vi "Convert_Midi_Data_To_Arduino.vi"() -> ()   [LabVIEW 2020]
uses:
  <vilib>/express/express arith-compare/Formula/XNode/ExpressFormulaBlockNode.xnode
panel:
  out "size(s)":i32
  out "String":string
  out "Array 3":dbl[](array[numeric])
  in  "Stop":bool
  out "x-y":dbl
  out "Array 2":i32[](array[numeric])
  out "Array":T1(array[cluster])
  out "value":T2(array[cluster])
  in  "JSON string":string
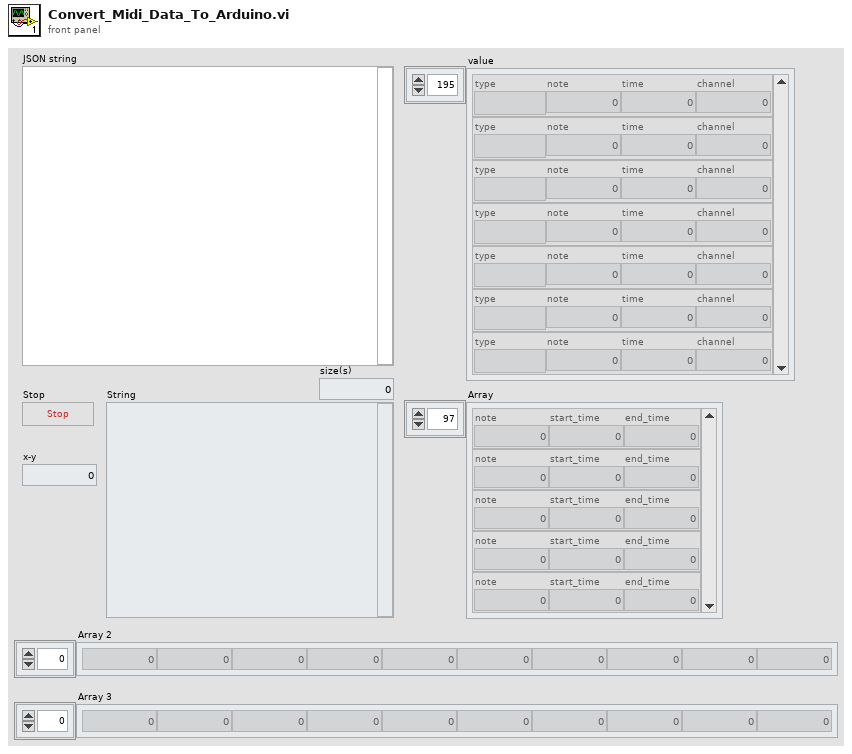
[diagram p1: front panel]
types:
  T1 = cluster{"note":i32, "start_time":u64, "end_time":u64}[]
  T2 = cluster{"type":string, "note":i32, "time":dbl, "channel":i32}[]
  T3 = cluster{"note":i32, "start_time":u64, "end_time":u64}
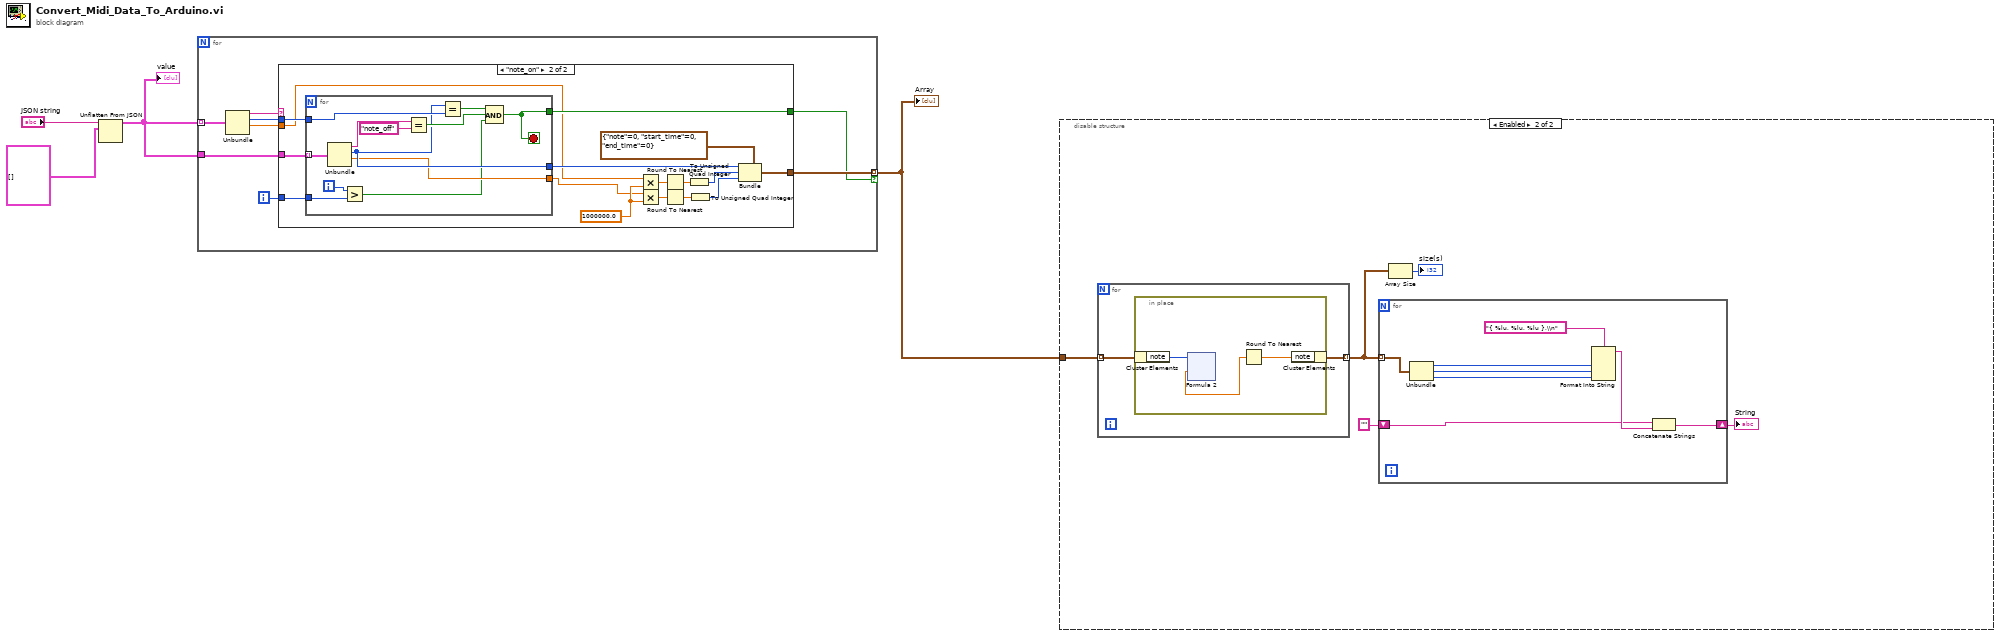
[diagram p0: block diagram]
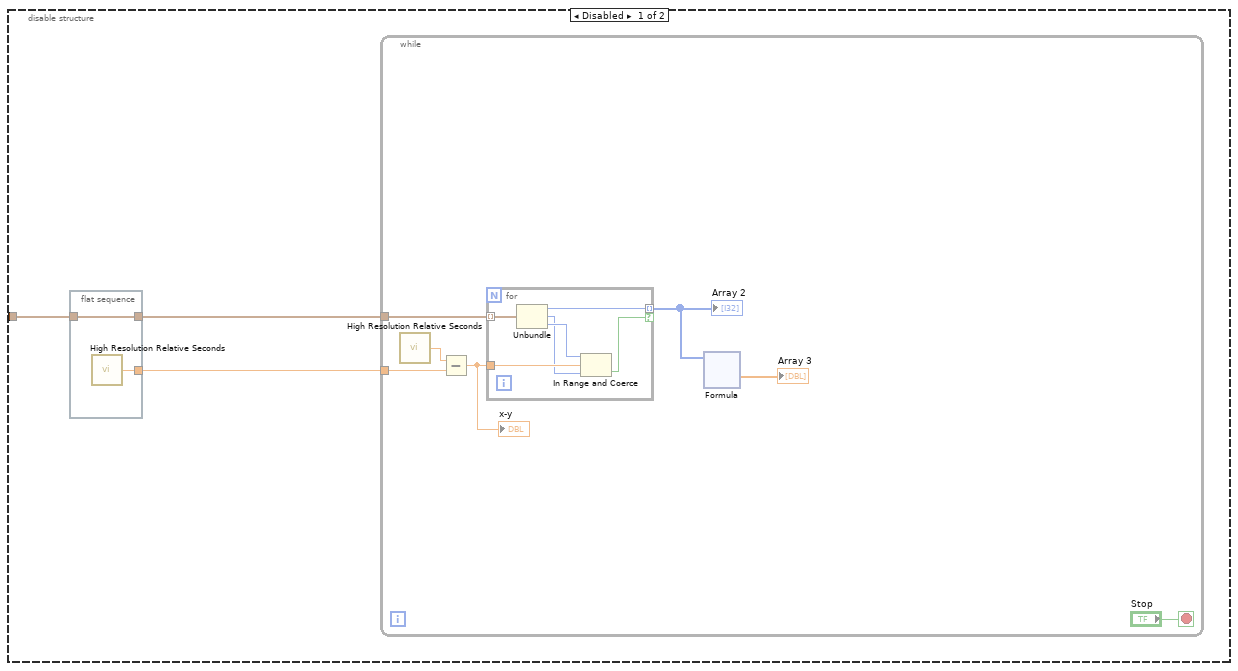
[diagram p2: hidden frame]
diagram:
  n1 = Unflatten From JSON(JSON string="JSON string", type and defaults=T2 []) -> (value=w2:T2)  [unwired: 5 in, 1 out]
  "value" <- w2
  n2 = for {
    tunnel: w2 -> [w12] mode=indexing
    tunnel: w2 -> [w10]
    tunnel: [w7] -> w1 mode=indexing if=w6
    i -> [w5]
    n3 = Unbundle(w12) -> ("type"=w11:string, "note"=w9:i32, "time"=w8:dbl)  [unwired: 1 out]
    n4 = case shown="\"note_on\"" w11 {
      tunnel: w10 -> [_ w28]
      tunnel: w9 -> [_ w27]
      tunnel: w8 -> [_ w16]
      tunnel: [_ w24] -> w7
      tunnel: [_ w23] -> w6
      tunnel: w5 -> [_ w22]
      frame Default {
      }
      frame "note_on" {
        w21 = 1000000.0 ("y")
        n5 = for {
          tunnel: w28 -> [w40] mode=indexing
          tunnel: w27 -> [w37]
          tunnel: [w34] -> w25
          tunnel: [w33] -> w15
          tunnel: [w32] -> w23
          tunnel: w22 -> [w30]
          i -> [w31]
          stop <- w32 stop-if-true
          n6 = Unbundle(w40) -> ("type"=w39:string, "note"=w34:i32, "time"=w33:dbl)  [unwired: 1 out]
          n7 = Greater?(x=w31, y=w30) -> (0:w29:bool)
          n8 = Equal?(x=w39, y="note_off") -> (x = y?=w35:bool)
          n9 = Equal?(x=w34, y=w37) -> (x = y?=w36:bool)
          n10 = Compound Arithmetic op=AND(w36, w35, w29) -> (w32:bool)
        }
        n11 = Multiply(x=w16, y=w21) -> (x*y=w20:dbl)
        n12 = Multiply(x=w15, y=w21) -> (x*y=w19:dbl)
        n13 = Round To Nearest(number=w20) -> (nearest integer value=w18:dbl)
        n14 = Round To Nearest(number=w19) -> (nearest integer value=w17:dbl)
        n15 = To Unsigned Quad Integer(1:w18) -> (0:w14:u64)
        n16 = To Unsigned Quad Integer(1:w17) -> (0:w13:u64)
        n17 = Bundle(cluster=T3 {"note"=0, "start_time"=0, "end_time"=0}, "note"=w25, "start_time"=w14, "end_time"=w13) -> (w24:T3)
      }
    }
  }
  "Array" <- w1
  n18 = disable-structure shown="Enabled" {
    disable-tunnel: w1 -> [w41 w73]
    frame Disabled {
      n19 = flat-sequence {
        tunnel: [w45] -> w43
        tunnel: [w44] -> w42
        tunnel: w41 -> [w44]
        frame #0 {
          n20 = call <vilib>:"High Resolution Relative Seconds.vi"() -> ("relative seconds"=w45:dbl)
        }
      }
      n21 = while {
        tunnel: w42 -> [w52]
        tunnel: w43 -> [w51]
        stop <- "Stop" stop-if-true
        n22 = call <vilib>:"High Resolution Relative Seconds.vi"() -> ("relative seconds"=w50:dbl)
        n23 = Subtract(x=w50, y=w51) -> (x-y=w49:dbl)
        "x-y" <- w49
        n24 = for {
          tunnel: w52 -> [w68] mode=indexing
          tunnel: w49 -> [w67]
          tunnel: [w64] -> w47 mode=indexing if=w63
          n25 = Unbundle(w68) -> ("note"=w64:i32, "start_time"=w65:u64, "end_time"=w66:u64)
          n26 = In Range and Coerce(upper limit=w66, x=w67, lower limit=w65) -> (In Range?=w63:bool)  [unwired: 1 out]
        }
        "Array 2" <- w47
        n27 = xnode "Formula"("X1"=w47) -> ("Result"=→"Array 3":dbl[])  [unwired: 1 in, 1 out]
      }
    }
    frame Enabled {
      n28 = for {
        tunnel: w73 -> [w83] mode=indexing
        tunnel: [w82] -> w70 mode=indexing
        n29 = in-place {
          n30 = in-place-cluster #1(w83) -> ("note"=w86:i32)
          n31 = xnode "Formula 2"("X1"=w86) -> ("Result"=w85:dbl)  [unwired: 1 in, 1 out]
          n32 = Round To Nearest(number=w85) -> (nearest integer value=w84:dbl)
          n33 = in-place-cluster #1("note"=w84) -> (w82:T3)
        }
      }
      n34 = for {
        tunnel: w70 -> [w80] mode=indexing
        shift-right: [w77] -> w71
        shift-left: "" -> [w76]
        n35 = Unbundle(w80) -> ("note"=w79:i32, "start_time"=w75:u64, "end_time"=w74:u64)
        n36 = Format Into String(format string="{ %lu, %lu, %lu },\\n", w79, w75, w74) -> (resulting string=w78:string)  [unwired: 2 in, 1 out]
        n37 = Concatenate Strings(w76, w78) -> (w77:string)
      }
      "String" <- w71
      n38 = Array Size(array=w70) -> (size(s)=→"size(s)":i32)
    }
  }
